vi "IndexaEstaticos.vi"(2 "Strings":string[][](array[string])) -> (16 "StringsIndexadas":string[][](array[string]))   [LabVIEW 2017]
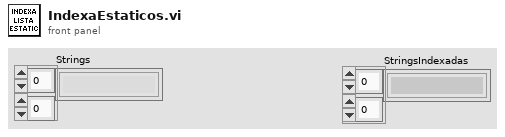
[diagram p1: front panel]
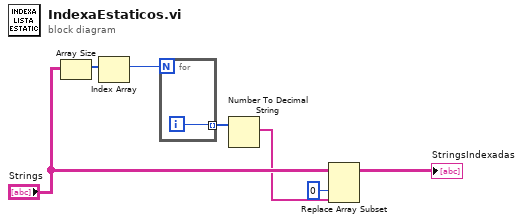
[diagram p0: block diagram]
diagram:
  n1 = Array Size(array="Strings") -> (size(s)=w7:i32[])
  n2 = Index Array(array=w7) -> (element=w6:i32)  [unwired: 1 in]
  n3 = for {
    N: w6 -> [_]
    tunnel: [w8] -> w5 mode=indexing
    i -> [w8]
  }
  n4 = Number To Decimal String(number=w5) -> (decimal integer string=w2:string[])  [unwired: 1 in]
  n5 = Replace Array Subset(array="Strings", new element=w2, index (col)=0 ("disabled index (col)")) -> (→"StringsIndexadas":string[][])  [unwired: 1 in]
